vi "GetConfig2.vi"(8 "error in (no error)":errorcluster, 11 "C37.118 PMU in":refnum<class "C37.118 PMU.lvclass">) -> (0 "error out":errorcluster, 3 "C37.118 PMU out":refnum<class "C37.118 PMU.lvclass">)   [LabVIEW 2018, in "SensorPlugins.lvlib" / "C37.118 PMU.lvclass"]
uses:
  C37.118 PMU.lvclass
  Typedef/eCmdTypes.ctl
  C37.118 PMU.lvclass/C37.118 PMU.ctl
  Accessors/Read CmdSocket.vi
  Accessors/Read PMUComms.vi
  <userlib>/NIST/Socket Class/Classes/Socket.Base/Socket.Base.lvclass
  PmuBaseClass/PmuBase.lvclass
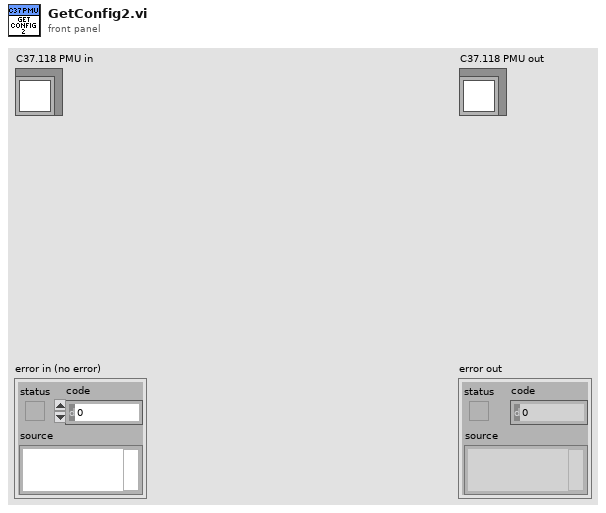
[diagram p1: front panel]
types:
  T1 = typedef "SensorPlugins.lvlib/C37.118 PMU.lvclass/eCmdTypes.ctl" = enum16{"Stop realtime data", "Start realtime data", "Send HDR file", "Send CFG-1 file", "Send CFG-2 file"}
  T2 = typedef "SensorPlugins.lvlib/C37.118 PMU.lvclass/PMUComms.ctl" = cluster{"PMU IP Address":string, "CMD Comms Type":T3, "Data Comms Type":T3, "CMD Port":u16, "Data Port":u16, "PMU ID":u16}
  T3 = typedef "SensorPlugins.lvlib/C37.118 PMU.lvclass/eCommsType.ctl" = enum16{"TCP", "UDP", "USB", "GPIB"}
  T4 = typedef "SensorPlugins.lvlib/PmuBase.lvclass/PMUDataType.ctl" = enum16{"undefined", "data", "header", "config 1", "config 2", "config 3", "command"}
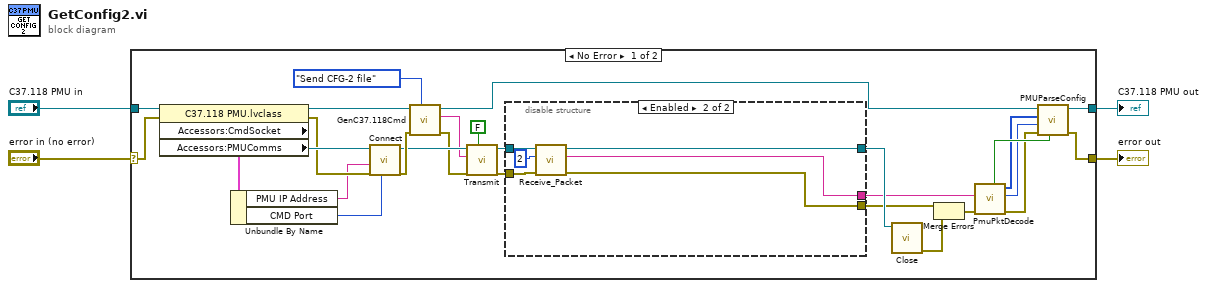
[diagram p0: block diagram]
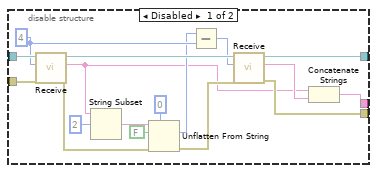
[diagram p2: hidden frame]
diagram:
  n1 = case shown="No Error" "error in (no error)" {
    selector: "error in (no error)" -> [w8 w57]
    tunnel: [w7 w57] -> w3
    tunnel: [w6 w56] -> w1
    tunnel: "C37.118 PMU in" -> [w9 w56]
    frame No Error {
      n2 = property class="C37.118 PMU.lvclass"(reference=w9, error in=w8) -> (reference out=w27:refnum<class "C37.118 PMU.lvclass">, error out=w30:errorcluster, "Accessors:CmdSocket"=w31:refnum<class "Socket.Base.lvclass">, "Accessors:PMUComms"=w32:T2)
      n3 = Unbundle By Name(w32) -> ("PMU IP Address"=w28:string, "CMD Port"=w29:u16)
      n4 = call-dynamic "Connect.vi"("remote_port"=w29, "error in (no error)"=w30, "remote_address"=w28, "Socket.Base in"=w31) -> ("error out"=w26:errorcluster, "Socket.Base out"=w24:refnum<class "Socket.Base.lvclass">)  [unwired: 6 in]
      n5 = call "GenC37.118Cmd.vi"("Function"=eCmdTypes."Send CFG-2 file", "error in (no error)"=w26, "PMUClass"=w27) -> ("error out"=w21:errorcluster, "Command"=w22:string, "PMUClass"=w5:refnum<class "C37.118 PMU.lvclass">)  [unwired: 6 in]
      n6 = call-dynamic "Transmit.vi"("packet? (f)"=FALSE, "error in (no error)"=w21, "data"=w22, "Socket.Base in"=w24) -> ("error out"=w19:errorcluster, "Socket.Base out"=w20:refnum<class "Socket.Base.lvclass">)  [unwired: 5 in, 1 out]
      n7 = disable-structure shown="Enabled" {
        disable-tunnel: w20 -> [w49 w54]
        disable-tunnel: w19 -> [w48 w55]
        disable-tunnel: [w42 w52] -> w12
        disable-tunnel: [w36 w50] -> w11
        disable-tunnel: [w33 w51] -> w10
        frame Disabled {
          w40 = u32 4 ("bufsize (0)")
          n8 = call-dynamic "Receive.vi"("error in (no error)"=w48, "bufsize (0)"=w40, "Socket.Base in"=w49) -> ("error out"=w44:errorcluster, "data_out"=w34:string, "Socket.Base out"=w43:refnum<class "Socket.Base.lvclass">)  [unwired: 5 in, 1 out]
          n9 = String Subset(string=w34, offset (0)=2) -> (substring=w46:string)  [unwired: 1 in]
          n10 = Unflatten From String(type=u16 0, binary string=w46, data includes array or string size? (T)=FALSE, error in (no error)=w44) -> (value=w39:u16, error out=w37:errorcluster)  [unwired: 1 in, 1 out]
          n11 = Subtract(x=w39, y=w40) -> (x-y=w38:u32)
          n12 = call-dynamic "Receive.vi"("error in (no error)"=w37, "bufsize (0)"=w38, "Socket.Base in"=w43) -> ("error out"=w36:errorcluster, "data_out"=w35:string, "Socket.Base out"=w42:refnum<class "Socket.Base.lvclass">)  [unwired: 5 in, 1 out]
          n13 = Concatenate Strings(w34, w35) -> (w33:string)
        }
        frame Enabled {
          n14 = call-dynamic "Receive_Packet.vi"("error in (no error)"=w55, "bufsize (0)"=u32 2, "Socket.Base in"=w54) -> ("error out"=w50:errorcluster, "data_out"=w51:string, "Socket.Base out"=w52:refnum<class "Socket.Base.lvclass">)  [unwired: 5 in, 1 out]
        }
      }
      n15 = call-dynamic "Close.vi"("Socket.Base in"=w12) -> ("error out"=w13:errorcluster)  [unwired: 9 in, 1 out]
      n16 = Merge Errors(w11, w13) -> (w14:errorcluster)
      n17 = call "PmuPktDecode.vi"("error in (no error)"=w14, "PktData"=w10) -> ("error out"=w15:errorcluster, "PMUDataType"=w16:T4, "PktData"=w17:u8[], "SyncOK"=w18:bool)  [unwired: 5 in, 1 out]
      n18 = call "PMUParseConfig.vi"("SyncOK"=w18, "error in (no error)"=w15, "PMUDataType"=w16, "PacketBodyIn"=w17, "C37.118 PMU.lvclass"=w5) -> ("error out"=w7:errorcluster, "C37.118 PMU.lvclass"=w6:refnum<class "C37.118 PMU.lvclass">)  [unwired: 5 in]
    }
    frame Error {
    }
  }
  "error out" <- w3
  "C37.118 PMU out" <- w1
